vi "HRR-Move.vi"(7 "N° motores":i32, 8 "error in":errorcluster, 10 "Pos, Vel":u16[][](array[numeric]), 11 "FPGA VI Reference In":refnum<k20>) -> (0 "error out":errorcluster, 3 "FPGA VI Reference Out":refnum<k20>)   [LabVIEW 2019]
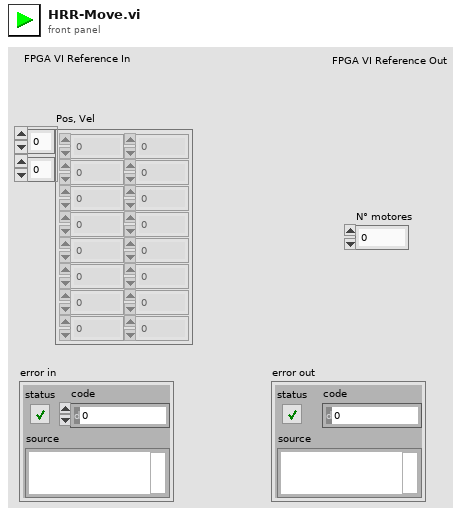
[diagram p1: front panel]
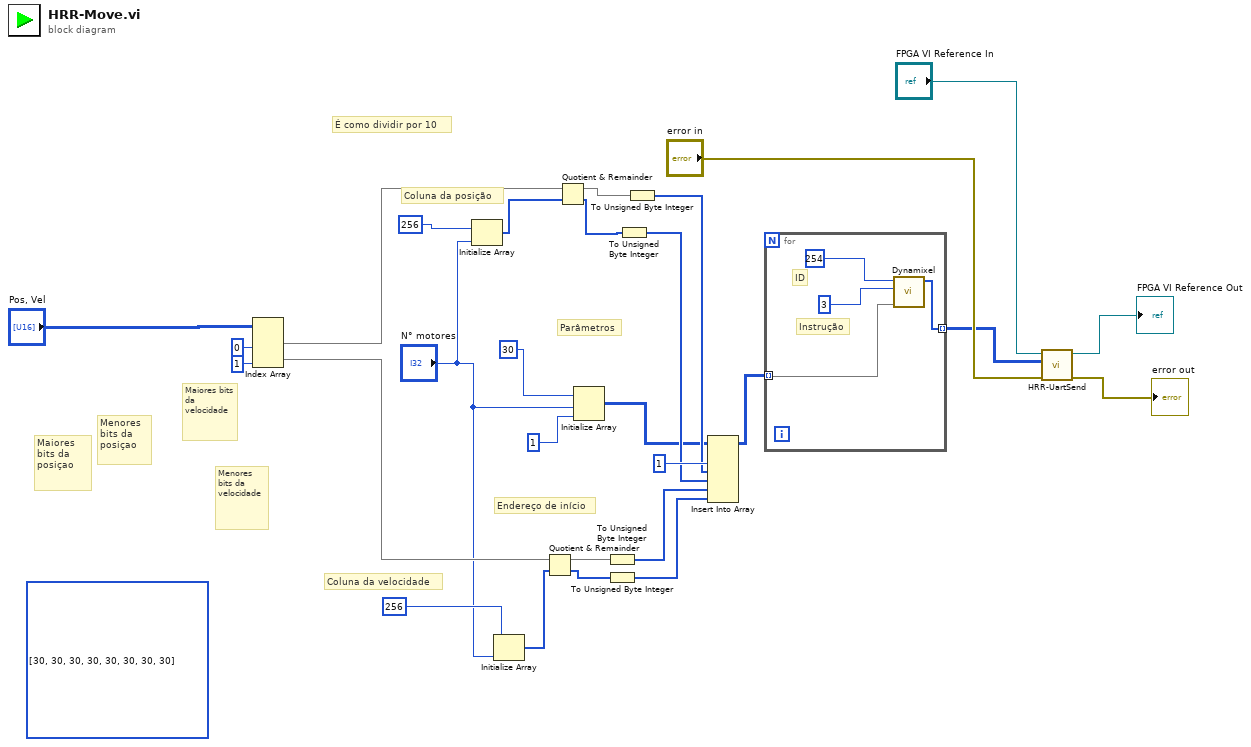
[diagram p0: block diagram]
diagram:
  (unwired) u8[][] [[30], [30], [30], [30], [30], [30], [30], [30]] ("array")
  # "Menores bits da velocidade"
  # "Maiores bits da velocidade"
  # "Menores bits da posiçao"
  # "Maiores bits da posiçao"
  # "É como dividir por 10"
  # "Coluna da velocidade"
  # "Coluna da posição"
  # "Parâmetros"
  # "Endereço de início"
  n1 = Index Array(array="Pos, Vel", index (col) #1=0 ("disabled index (col)"), index (col) #2=1 ("index (col)")) -> (element #1=w15:u16[], element #2=w14:u16[])  [unwired: 2 in]
  n2 = Initialize Array(u16 256, "N° motores") -> (w4:u16[])
  n3 = Initialize Array(u16 256, "N° motores") -> (w6:u16[])
  n4 = Quotient & Remainder(x=w14, y=w6) -> (x-y*floor(x/y)=w20:u16[], floor(x/y)=w19:u16[])
  n5 = Quotient & Remainder(x=w15, y=w4) -> (x-y*floor(x/y)=w25:u16[], floor(x/y)=w23:u16[])
  n6 = Initialize Array(u8 30, "N° motores", 1 ("dimension size")) -> (w1:u8[][])
  n7 = To Unsigned Byte Integer(number=w20) -> (unsigned 8bit integer=w18:u8[])
  n8 = To Unsigned Byte Integer(number=w19) -> (unsigned 8bit integer=w17:u8[])
  n9 = To Unsigned Byte Integer(number=w23) -> (unsigned 8bit integer=w22:u8[])
  n10 = To Unsigned Byte Integer(number=w25) -> (unsigned 8bit integer=w24:u8[])
  n11 = Insert Into Array(array=w1, index (col)=1 ("disabled index (col)"), new element #1=w24, new element #2=w22, new element #3=w18, new element #4=w17) -> (w21:u8[][])  [unwired: 1 in]
  n12 = for {
    tunnel: w21 -> [w30] mode=indexing
    tunnel: [w29] -> w9 mode=indexing
    # "Instrução"
    # "ID"
    n13 = call "Dynamixel.vi"("ID"=u8 254, "Instruction"=u8 3, "Array in"=w30) -> ("Array out"=w29:u8[])  [unwired: 7 in]
  }
  n14 = call "HRR-UartSend.vi"("error in (no error)"="error in", "Array"=w9, "Refnum in"="FPGA VI Reference In") -> ("error out"=→"error out":errorcluster, "Refnum out"=→"FPGA VI Reference Out":refnum<k20>)  [unwired: 7 in]
